vi "Update Value.vi"(6 "Time":dbl, 8 "error in (no error)":errorcluster, 11 "SimpleChart in":refnum<class "SimpleChart.lvclass">) -> (0 "error out":errorcluster, 1 "Update":bool, 2 "Value":variant, 3 "SimpleChart out":refnum<class "SimpleChart.lvclass">)   [LabVIEW 2020, in "VolatusGUIElements.lvlib" / "SimpleChart.lvclass"]
uses:
  SimpleChart.lvclass
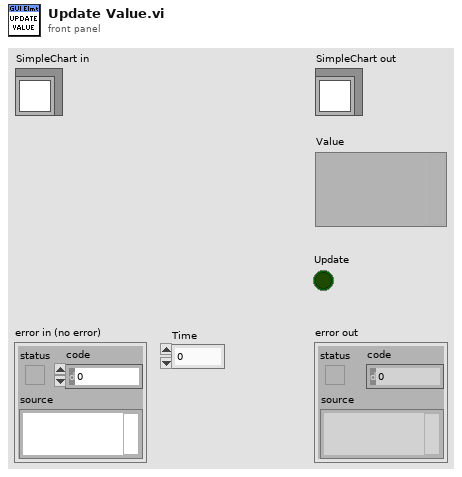
[diagram p1: front panel]
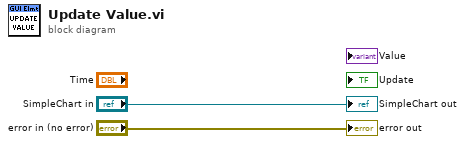
[diagram p0: block diagram]
diagram:
  "error out" <- "error in (no error)"
  "SimpleChart out" <- "SimpleChart in"
